vi "Update Status.vi"(6 "Error In":errorcluster, 7 "Status Limit":i32, 8 "Status History In":string[](array[string]), 9 "Application In":refnum<class "Application.lvclass">) -> (0 "Error Out":errorcluster, 1 "Status":string, 2 "Status History Out":string[](array[string]), 3 "Application Out":refnum<class "Application.lvclass">)   [LabVIEW 2023, in "Application.lvclass"]
doc: "The VI adds the current status to the status history and converts it to string to display"
uses:
  Application.lvclass
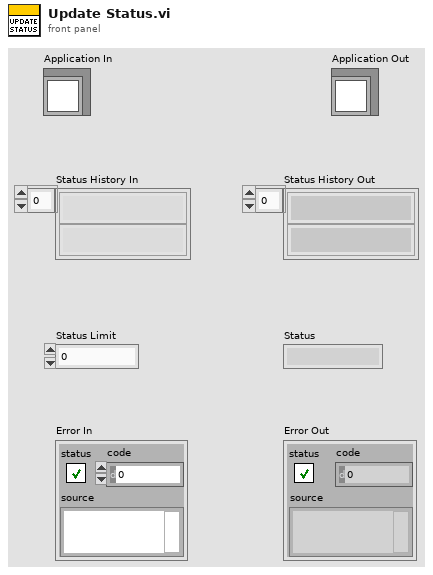
[diagram p1: front panel]
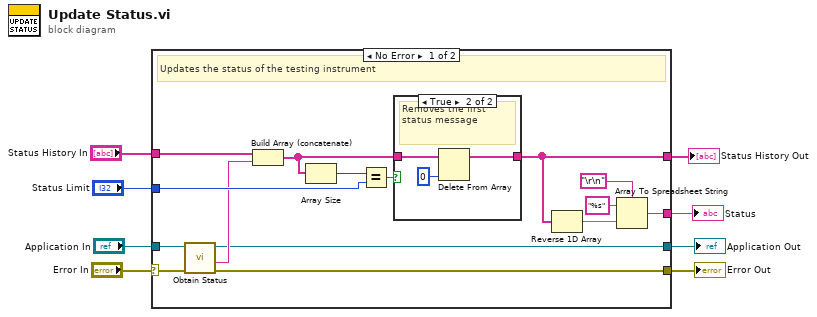
[diagram p0: block diagram]
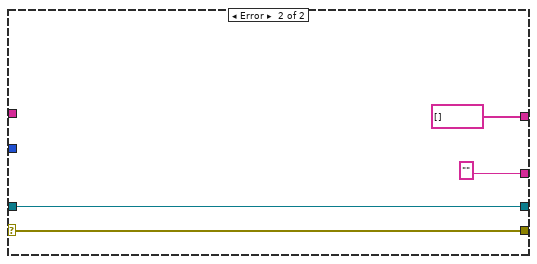
[diagram p3: hidden frame]
diagram:
  n1 = case shown="No Error" "Error In" {
    selector: "Error In" -> [w15 w31]
    tunnel: [w14 w31] -> w7
    tunnel: "Status History In" -> [w20 _]
    tunnel: "Status Limit" -> [w19 _]
    tunnel: "Application In" -> [w12 w30]
    tunnel: [w11 w30] -> w3
    tunnel: [w10 "" ("spreadsheet string")] -> w2
    tunnel: [w9 string[] []] -> w1
    frame No Error {
      # "Updates the status of the testing instrument"
      n2 = call-dynamic "Obtain Status.vi"("Error In"=w15, "Application In"=w12) -> ("Error Out"=w14:errorcluster, "Status"=w13:string, "Application Out"=w11:refnum<class "Application.lvclass">)  [unwired: 6 in, 1 out]
      n3 = Build Array (concatenate)(w20, w13) -> (w23:string[])
      n4 = Array Size(array=w23) -> (size(s)=w22:i32)
      n5 = Equal?(x=w22, y=w19) -> (x = y?=w21:bool)
      n6 = case shown="True" w21 {
        tunnel: w23 -> [w24 w27]
        tunnel: [w24 w25] -> w9
        frame False {
        }
        frame True {
          # "Removes the first status message"
          n7 = Delete From Array(array=w27, index=0) -> (array with subset deleted=w25:string[])  [unwired: 1 in, 1 out]
        }
      }
      n8 = Reverse 1D Array(array=w9) -> (reversed array=w18:string[])
      n9 = Array To Spreadsheet String(delimiter (Tab)="\r\n", array=w18, 3:"%s" ("format string")) -> (spreadsheet string=w10:string)
    }
    frame Error {
    }
  }
  "Error Out" <- w7
  "Application Out" <- w3
  "Status" <- w2
  "Status History Out" <- w1
